vi "Msg.vi"(7 "jettl in":refnum<class "jettl.lvclass">, 11 "Last Ack Msg Strategy in":refnum<class "Last Ack Msg Strategy.lvclass">) -> (5 "jettl out":refnum<class "jettl.lvclass">)   [LabVIEW 2021, in "jettl.lvlib" / "Last Ack Msg Strategy.lvlib" / "Last Ack Msg Strategy.lvclass"]
uses:
  Last Ack Msg Strategy.lvclass
  jettl/jettl.lvclass
  Last Ack/Last Ack.lvclass
  Last Ack Msg Strategy.lvclass/Last Ack Msg Strategy.ctl
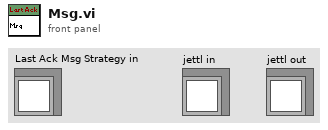
[diagram p1: front panel]
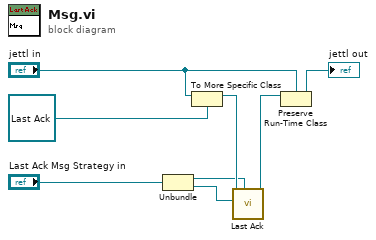
[diagram p0: block diagram]
diagram:
  n1 = Unbundle "Unbundle"("Last Ack Msg Strategy in") -> (w1:refnum<class "Sender.lvclass">, w2:refnum<class "jettl.lvclass">)
  n2 = To More Specific Class(target class=refnum<class "Last Ack.lvclass"> refnum ("jettl.lvlib:jettl Msg Last Ack Creator Queue.lvlib:jettl Msg Last Ack Creator Queue.lvclass"), reference="jettl in") -> (specific class reference=w4:refnum<class "Last Ack.lvclass">)  [unwired: 1 in, 1 out]
  n3 = call-dynamic "Last Ack.vi"("Sender"=w1, "jettl"=w2, "Last Ack in"=w4) -> ("Last Ack out"=w3:refnum<class "Last Ack.lvclass">)  [unwired: 8 in]
  n4 = Preserve Run-Time Class(object in=w3, 2:"jettl in") -> (object out=→"jettl out":refnum<class "jettl.lvclass">)  [unwired: 1 in, 1 out]
